vi "loadDataPerChannel.vi"(8 "error in (no error)":errorcluster, 10 "data":dbl[][][](array[numeric]), 11 "K2602 in":refnum<class "K2602.lvclass">) -> (0 "error out":errorcluster, 3 "K2602 out":refnum<class "K2602.lvclass">)   [LabVIEW 2011, in "Hardware.lvlib" / "Channels.lvlib" / "K2602.lvclass"]
uses:
  K2602.lvclass
  K2602.lvclass/K2602.ctl
  Tools/Filing/FileSystem/FileSystem.lvclass
  Channels.lvlib
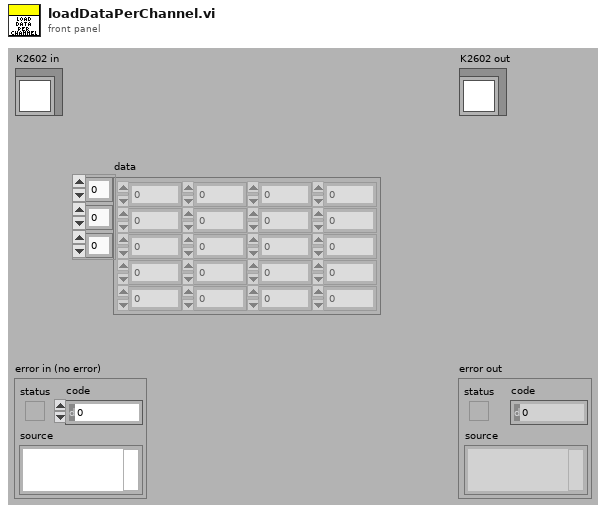
[diagram p1: front panel]
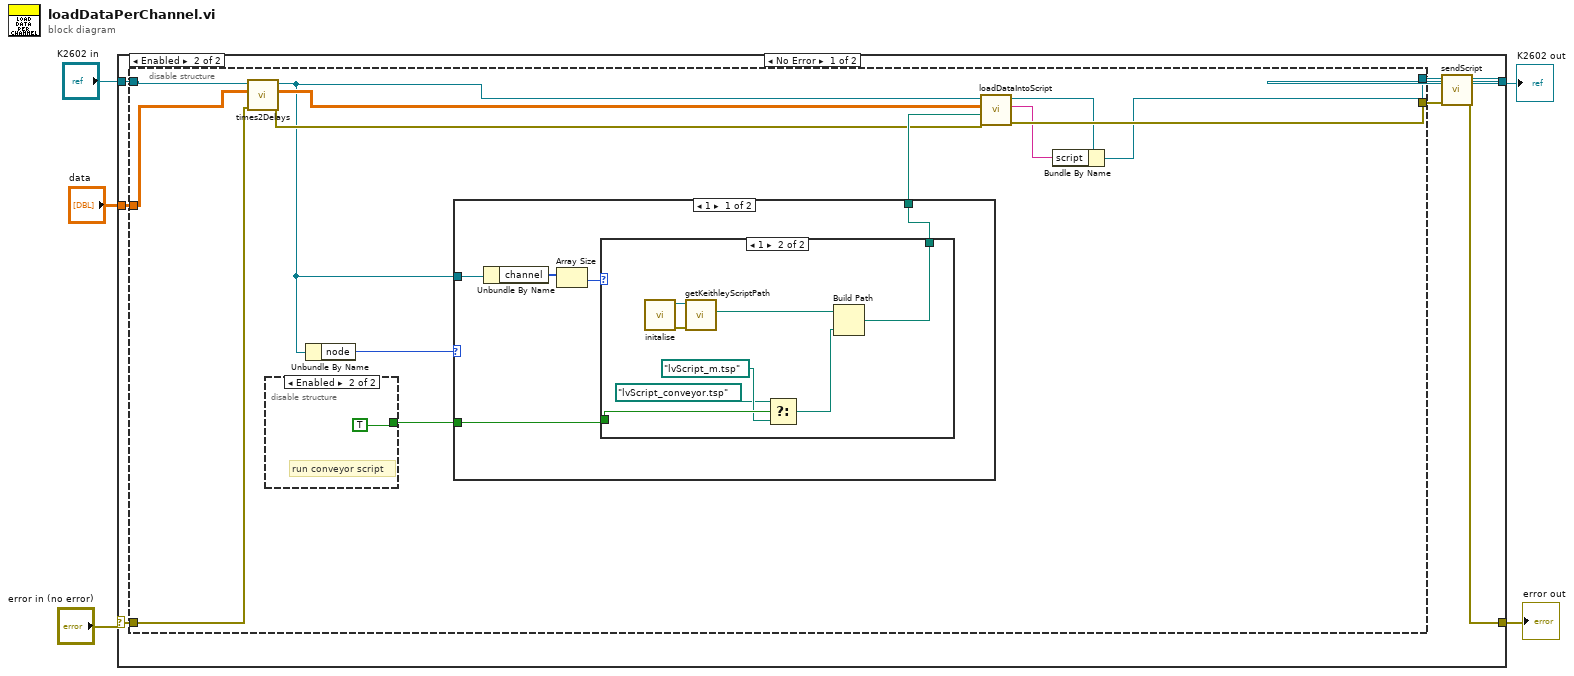
[diagram p0: block diagram]
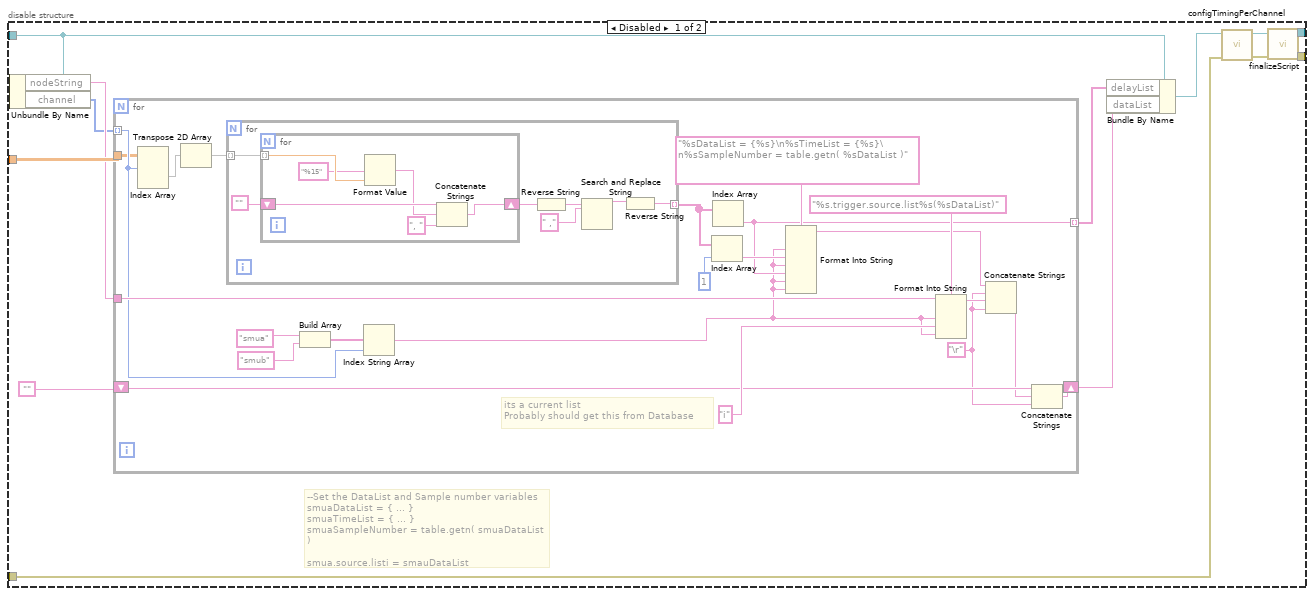
[diagram p2: hidden frame]
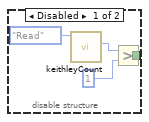
[diagram p3: hidden frame]
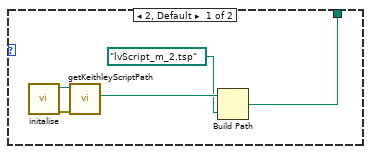
[diagram p4: hidden frame]
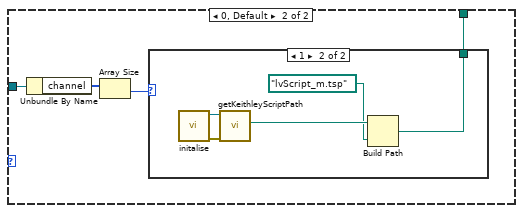
[diagram p5: hidden frame]
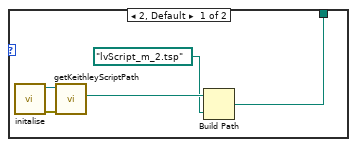
[diagram p6: hidden frame]
diagram:
  n1 = case shown="No Error" "error in (no error)" {
    selector: "error in (no error)" -> [w10 w111]
    tunnel: [w6 w111] -> w4
    tunnel: [w7 w112] -> w2
    tunnel: "K2602 in" -> [w11 w112]
    tunnel: "data" -> [w12 _]
    frame No Error {
      n2 = disable-structure shown="Enabled" {
        disable-tunnel: w12 -> [w25 w67]
        disable-tunnel: w11 -> [w23 w68]
        disable-tunnel: w10 -> [w18 w66]
        disable-tunnel: [w15 w69] -> w9
        disable-tunnel: [w14 w73] -> w8
        frame Disabled {
          # "--Set the DataList and Sample number variables\nsmuaDataList = { ... }\nsmuaTimeList = { ... }\nsmuaSampleNumber = table.getn( smuaDataList ) \n\nsmua.source.listi = smauDataList"
          n3 = Unbundle By Name(w23) -> ("nodeString"=w24:string, "channel"=w13:i32[])
          n4 = for {
            tunnel: w25 -> [w28]
            tunnel: w24 -> [w44]
            tunnel: [w32] -> w22 mode=indexing
            shift-right: [w39] -> w20
            shift-left: "" -> [w38]
            tunnel: w13 -> [w29] mode=indexing
            w30 = "\r"
            # "its a current list\nProbably should get this from Database"
            n5 = Index Array(array=w28, index (dim 0)=w29) -> (element=w27:dbl[][])  [unwired: 2 in]
            n6 = Transpose 2D Array(2D array=w27) -> (transposed array=w31:dbl[][])
            n7 = for {
              tunnel: w31 -> [w54] mode=indexing
              tunnel: [w48] -> w40 mode=indexing
              n8 = for {
                tunnel: w54 -> [w60] mode=indexing
                shift-right: [w55] -> w52
                shift-left: "" -> [w58]
                n9 = Format Value(format string="%15", value (0)=w60) -> (output string=w57:string)  [unwired: 1 in]
                n10 = Concatenate Strings(w58, w57, ", ") -> (w55:string)
              }
              n11 = Reverse String(1:w52) -> (0:w51:string)
              n12 = Search and Replace String(input string=w51, search string=" ,") -> (result string=w49:string)  [unwired: 6 in, 3 out]
              n13 = Reverse String(1:w49) -> (0:w48:string)
            }
            n14 = Build Array("smua", "smub") -> (w45:string[])
            n15 = Index String Array(1:w29, 2:w45) -> (0:w26:string)  [unwired: 1 in]
            n16 = Index Array(array=w40, index=1) -> (element=w36:string)
            n17 = Index Array(array=w40) -> (element=w32:string)  [unwired: 1 in]
            n18 = Format Into String(format string="%sDataList = {%s}\n%sTimeList = {%s}\n%sSampleNumber = table.getn( %sDataList )", w26, w36, w26, w32, w26, w26) -> (resulting string=w34:string)  [unwired: 2 in, 1 out]
            n19 = Format Into String(format string="%s.trigger.source.list%s(%sDataList)", initial string=w44, w26, "i", w26) -> (resulting string=w33:string)  [unwired: 1 in, 1 out]
            n20 = Concatenate Strings(w34, w30, w33, w30) -> (w37:string)
            n21 = Concatenate Strings(w38, w37, w30) -> (w39:string)
          }
          n22 = Bundle By Name(cluster=w23, "delayList"=w22, "dataList"=w20) -> (w19:refnum<class "K2602.lvclass">)
          n23 = call-dynamic "configTimingPerChannel.vi"("error in (no error)"=w18, "K2602 in"=w19) -> ("error out"=w16:errorcluster, "K2602 out"=w17:refnum<class "K2602.lvclass">)  [unwired: 8 in]
          n24 = call "finalizeScript.vi"("error in (no error)"=w16, "K2602 in"=w17) -> ("error out"=w14:errorcluster, "K2602 out"=w15:refnum<class "K2602.lvclass">)  [unwired: 7 in, 1 out]
        }
        frame Enabled {
          n25 = call "times2Delays.vi"("error in (no error)"=w66, "data"=w67, "K2602 in"=w68) -> ("error out"=w65:errorcluster, "data out"=w64:dbl[][][], "K2602 out"=w63:refnum<class "K2602.lvclass">)  [unwired: 6 in]
          n26 = disable-structure shown="Enabled" {
            disable-tunnel: [w74 TRUE] -> w61
            frame Disabled {
              n27 = call "keithleyCount.vi"("Action"=enum16{"Read", "increment", "deincrement"}."Read") -> ("Numeric"=w76:i32)  [unwired: 10 in]
              n28 = Greater?(x=w76, y=1) -> (0:w74:bool)
            }
            frame Enabled {
              # "run conveyor script"
            }
          }
          n29 = Unbundle By Name(w63) -> ("node"=w62:i8)
          n30 = case shown="1" w62 {
            tunnel: [w83 w100] -> w72
            tunnel: w63 -> [w81 w98]
            tunnel: w61 -> [w79 _]
            frame 1 {
              n31 = Unbundle By Name(w81) -> ("channel"=w82:i32[])
              n32 = Array Size(array=w82) -> (size(s)=w80:i32)
              n33 = case shown="1" w80 {
                tunnel: [w84 w93] -> w83
                tunnel: w79 -> [_ w92]
                frame 2, Default {
                  n34 = call "initalise.vi"() -> ("error out"=w87:errorcluster, "FileSystem out"=w88:refnum<class "FileSystem.lvclass">)  [unwired: 10 in]
                  n35 = call "getKeithleyScriptPath.vi"("error in (no error)"=w87, "FileSystem in"=w88) -> ("keithleyScriptPath"=w86:path)  [unwired: 7 in, 2 out]
                  n36 = Build Path(base path=w86, name or relative path=path "lvScript_m_2.tsp" ("Path")) -> (appended path=w84:path)
                }
                frame 1 {
                  n37 = call "initalise.vi"() -> ("error out"=w95:errorcluster, "FileSystem out"=w96:refnum<class "FileSystem.lvclass">)  [unwired: 10 in]
                  n38 = call "getKeithleyScriptPath.vi"("error in (no error)"=w95, "FileSystem in"=w96) -> ("keithleyScriptPath"=w94:path)  [unwired: 7 in, 2 out]
                  n39 = Select(t=path "lvScript_conveyor.tsp" ("Path"), s=w92, f=path "lvScript_m.tsp" ("Path")) -> (s? t:f=w90:path)
                  n40 = Build Path(base path=w94, name or relative path=w90) -> (appended path=w93:path)
                }
              }
            }
            frame 0, Default {
              n41 = Unbundle By Name(w98) -> ("channel"=w99:i32[])
              n42 = Array Size(array=w99) -> (size(s)=w97:i32)
              n43 = case shown="1" w97 {
                tunnel: [w101 w106] -> w100
                frame 2, Default {
                  n44 = call "initalise.vi"() -> ("error out"=w104:errorcluster, "FileSystem out"=w105:refnum<class "FileSystem.lvclass">)  [unwired: 10 in]
                  n45 = call "getKeithleyScriptPath.vi"("error in (no error)"=w104, "FileSystem in"=w105) -> ("keithleyScriptPath"=w103:path)  [unwired: 7 in, 2 out]
                  n46 = Build Path(base path=w103, name or relative path=path "lvScript_m_2.tsp" ("Path")) -> (appended path=w101:path)
                }
                frame 1 {
                  n47 = call "initalise.vi"() -> ("error out"=w109:errorcluster, "FileSystem out"=w110:refnum<class "FileSystem.lvclass">)  [unwired: 10 in]
                  n48 = call "getKeithleyScriptPath.vi"("error in (no error)"=w109, "FileSystem in"=w110) -> ("keithleyScriptPath"=w108:path)  [unwired: 7 in, 2 out]
                  n49 = Build Path(base path=w108, name or relative path=path "lvScript_m.tsp" ("Path")) -> (appended path=w106:path)
                }
              }
            }
          }
          n50 = call "loadDataIntoScript.vi"("error in (no error)"=w65, "Path"=w72, "data"=w64, "K2602 in"=w63) -> ("error out"=w73:errorcluster, "script"=w71:string, "K2602 out"=w70:refnum<class "K2602.lvclass">)  [unwired: 5 in]
          n51 = Bundle By Name(cluster=w70, "script"=w71) -> (w69:refnum<class "K2602.lvclass">)
        }
      }
      n52 = call "sendScript.vi"("error in (no error)"=w8, "K2602 in"=w9) -> ("error out"=w6:errorcluster, "K2602 out"=w7:refnum<class "K2602.lvclass">)  [unwired: 8 in]
    }
    frame Error {
    }
  }
  "error out" <- w4
  "K2602 out" <- w2
